vi "GetWvl.vi"(0 "Visa Session":refnum<visa-resource-name>, 1 "error in (no error)":errorcluster) -> (2 "dup Visa Session":refnum<visa-resource-name>, 3 "strings array":string[](array[string]), 4 "symbol array":i32[](array[numeric]), 5 "error out":errorcluster)   [LabVIEW 2012]
panel:
  out "current wavelength":string
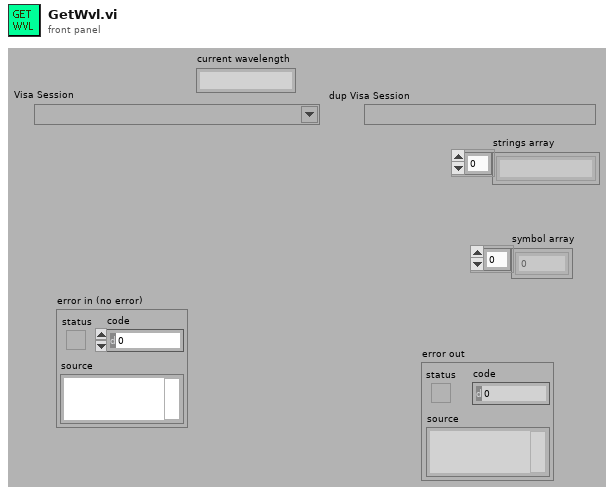
[diagram p1: front panel]
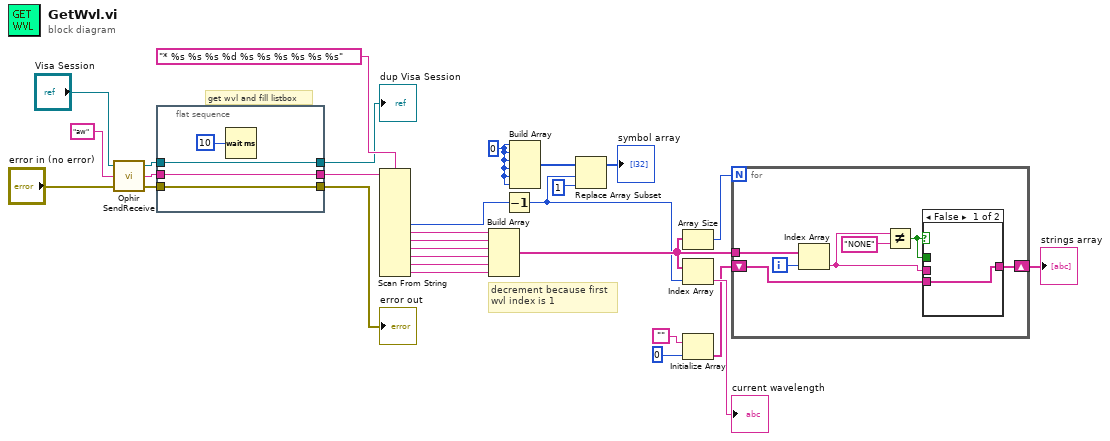
[diagram p0: block diagram]
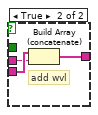
[diagram p2: hidden frame]
diagram:
  w12 = 0
  # "decrement because first wvl index is 1"
  # "get wvl and fill listbox"
  n1 = call "Ophir SendReceive.vi"("error in (no error)"="error in (no error)", "Command"="aw", "Visa Session"="Visa Session") -> ("error out"=w3:errorcluster, "Frame Output"=w5:string, "dup Visa Session"=w1:refnum<visa-resource-name>)
  n2 = flat-sequence {
    tunnel: [w32] -> w6
    tunnel: w5 -> [w32]
    tunnel: [w31] -> w4
    tunnel: w3 -> [w31]
    tunnel: [w30] -> w2
    tunnel: w1 -> [w30]
    frame #0 {
      n3 = Wait (ms)(milliseconds to wait=u32 10) -> ()  [unwired: 1 out]
    }
  }
  n4 = Scan From String "Scan From String"(format string="* %s %s %s %d %s %s %s %s %s %s", input string=w6) -> (output 4=w21:i32, output 5=w27:string, output 6=w26:string, output 7=w25:string, output 8=w24:string, output 9=w23:string, output 10=w22:string)  [unwired: 15 in, 3 out]
  n5 = Build Array(w27, w26, w25, w24, w23, w22) -> (w18:string[])
  n6 = Decrement(x=w21) -> (x-1=w8:i32)
  n7 = Build Array(w12, w12, w12, w12, w12, w12) -> (w11:i32[])
  n8 = Replace Array Subset(array=w11, new element=1 ("new element/subarray"), index=w8) -> (→"symbol array":i32[])
  n9 = Array Size(array=w18) -> (size(s)=w19:i32)
  n10 = Index Array(array=w18, index=w8) -> (element=→"current wavelength":string)
  n11 = Initialize Array("", 0) -> (w15:string[])
  n12 = for {
    N: w19 -> [_]
    shift-right: [w37] -> w7
    shift-left: w15 -> [w35]
    tunnel: w18 -> [w34]
    i -> [w40]
    n13 = Index Array(array=w34, index=w40) -> (element=w36:string)
    n14 = Not Equal?(x=w36, y="NONE") -> (x != y?=w38:bool)
    n15 = case shown="False" w38 {
      tunnel: w38 -> [_ _]
      tunnel: [w41 w44] -> w37
      tunnel: w36 -> [_ w42]
      tunnel: w35 -> [w41 w43]
      frame False {
      }
      frame True {
        # "add wvl"
        n16 = Build Array (concatenate)(w43, w42) -> (w44:string[])
      }
    }
  }
  "strings array" <- w7
  "dup Visa Session" <- w2
  "error out" <- w4
